vi "Untitled 5.vi"(2 "Camera Device  IN":T2, 3 "Camera Parameters":refnum<vi>, 4 "Selector":refnum<vi>, 5 "Stream?":refnum<vi>) -> (0 "Stream? OUT":bool, 1 "Camera Device OUT":T1)   [LabVIEW 2010]
uses:
  <vilib>/addons/PixeLINK/Low Level Functions/CAMERA_FEATURES.llb/TDPU-CameraFeatures-PixelFormat.ctl
  <vilib>/addons/PixeLINK/Low Level Functions/CAMERA_FEATURES.llb/TDPU-CameraFeatures-FeatureFlags.ctl
  <vilib>/addons/PixeLINK/Low Level Functions/CAMERA_FEATURES.llb/TDPU-CameraFeatures-FeatureIds.ctl
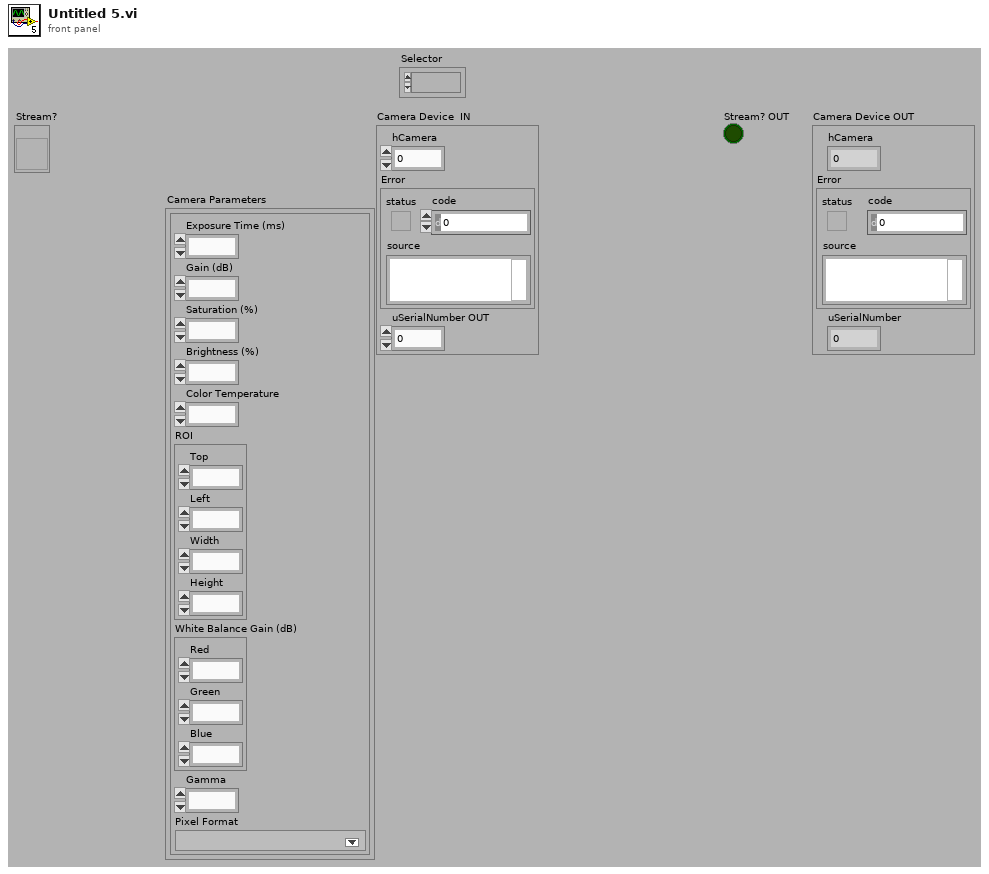
[diagram p1: front panel]
types:
  T1 = cluster{"hCamera":u32, "Error":errorcluster, "uSerialNumber":u32}
  T2 = cluster{"hCamera":u32, "Error":errorcluster, "uSerialNumber OUT":u32}
  T3 = typedef "TDPU-CameraFeatures-PixelFormat.ctl" = u16
  T4 = cluster{"Selector":u16, "Stream?":bool, "Camera Parameters":cluster{"Exposure Time (ms)":u32, "Gain (dB)":dbl, "Saturation (%)":dbl, "Brightness (%)":dbl, "Color Temperature":dbl, "ROI":cluster{"Top":i32, "Left":i32, "Width":i32, "Height":i32}, "White Balance Gain (dB)":cluster{"Red":dbl, "Green":dbl, "Blue":dbl}, "Gamma":dbl, "Pixel Format":T3}}
  T5 = cluster{"Exposure Time (ms)":u32, "Gain (dB)":dbl, "Saturation (%)":dbl, "Brightness (%)":dbl, "Color Temperature":dbl, "ROI":cluster{"Top":i32, "Left":i32, "Width":i32, "Height":i32}, "White Balance Gain (dB)":cluster{"Red":dbl, "Green":dbl, "Blue":dbl}, "Gamma":dbl, "Pixel Format":T3}
  T6 = cluster{"Exposure Time (ms)":dbl, "Gain (dB)":dbl, "Saturation (%)":dbl, "Brightness (%)":dbl, "Color Temperature":dbl, "ROI":cluster{"Top":i32, "Left":i32, "Width":i32, "Height":i32}, "White Balance Gain (dB)":cluster{"Red":dbl, "Green":dbl, "Blue":dbl}, "Gamma":dbl, "Pixel Format":T3}
  T7 = enum16{"Exposure Time (ms)", "Gain (dB)", "Saturation (%)", "Brightness (%)", "Color Temperature (%)", "ROI", "White Balance Gain (dB)", "Gamma", "Pixel Format", "Selector", "Stream", "Nothing"}[]
  T8 = typedef "TDPU-CameraFeatures-FeatureFlags.ctl" = u32
  T9 = typedef "TDPU-CameraFeatures-FeatureIds.ctl" = u32
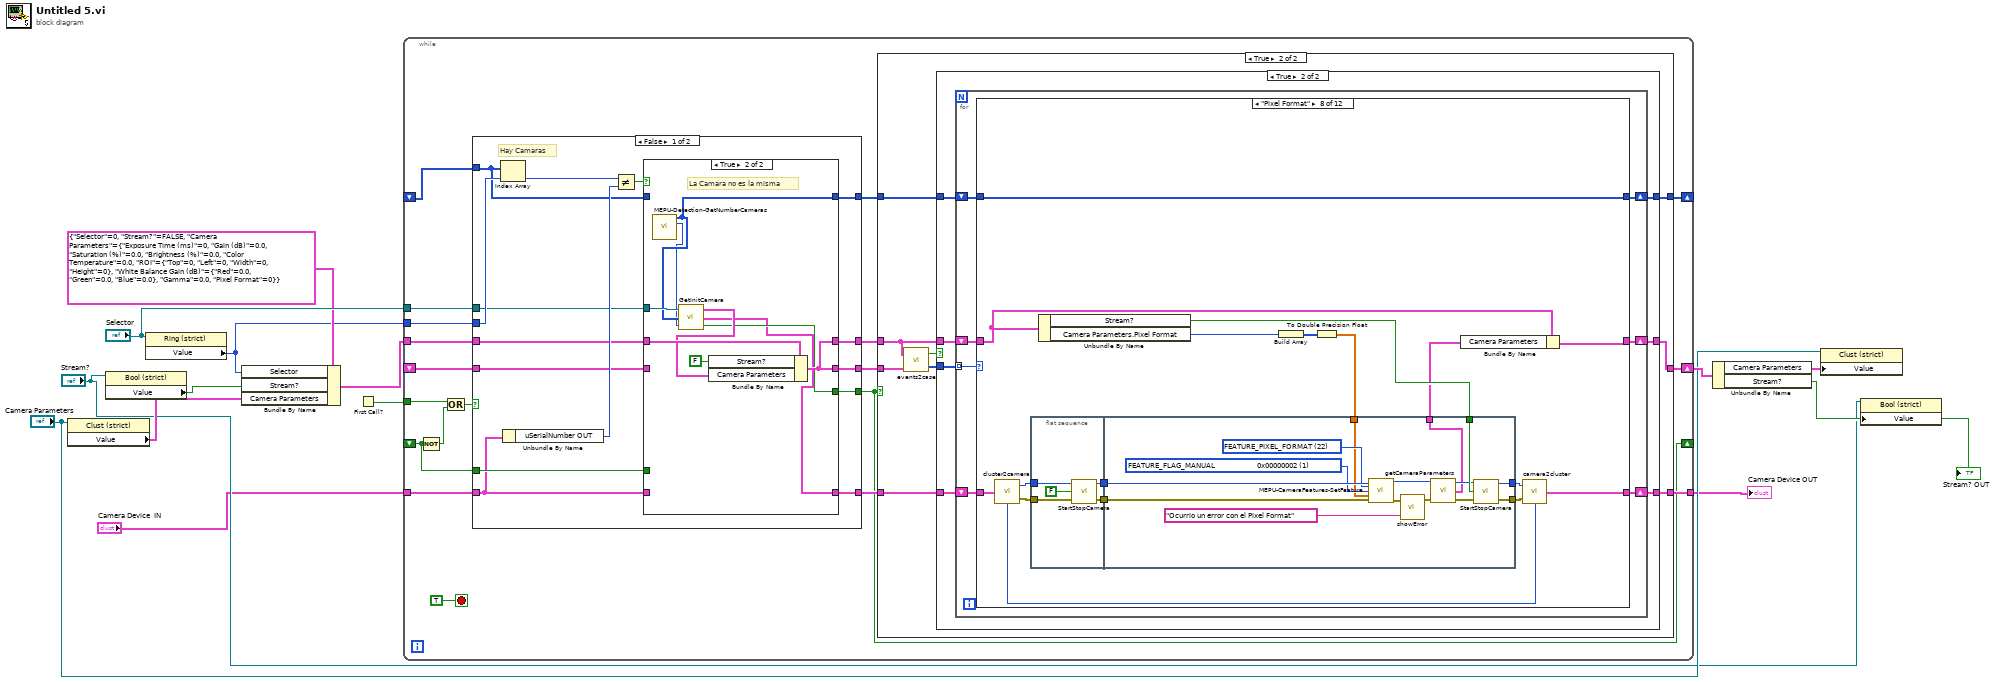
[diagram p0: block diagram]
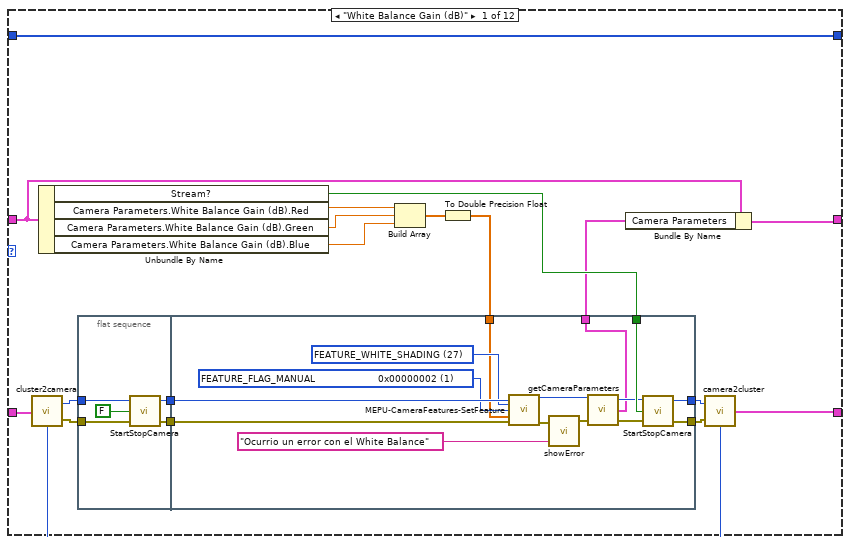
[diagram p4: hidden frame]
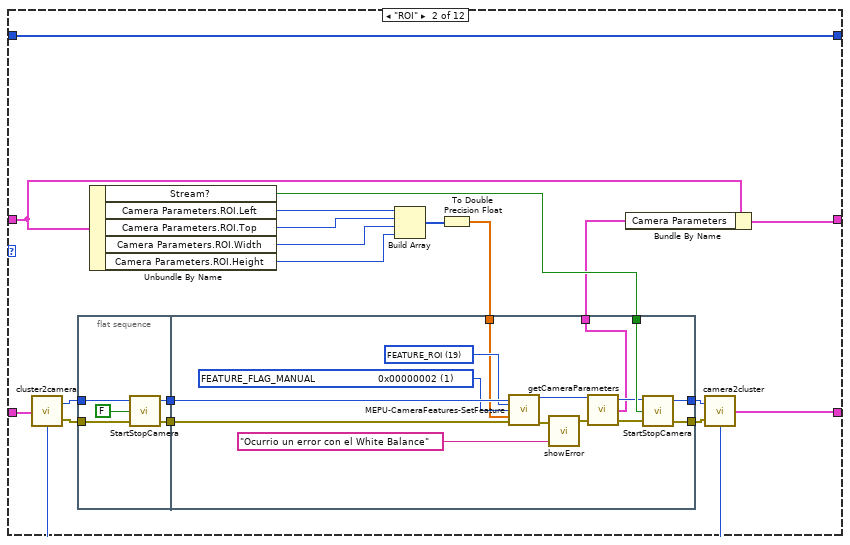
[diagram p5: hidden frame]
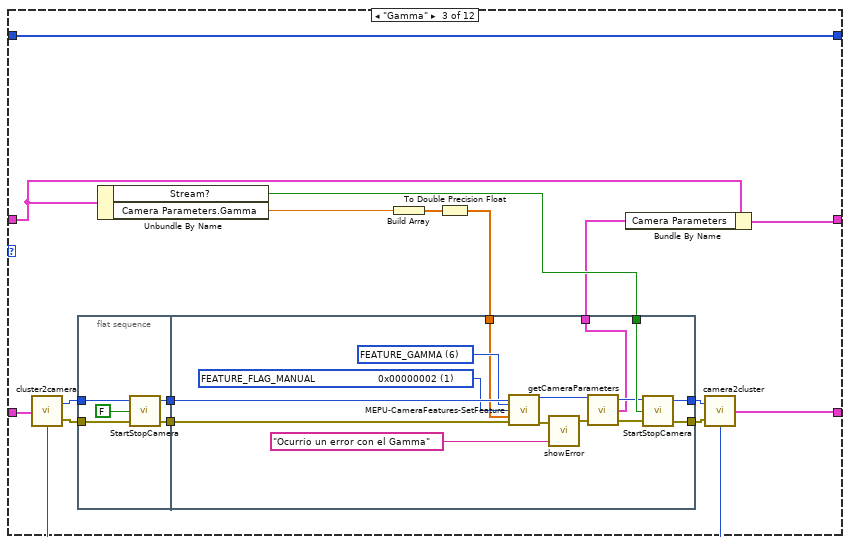
[diagram p6: hidden frame]
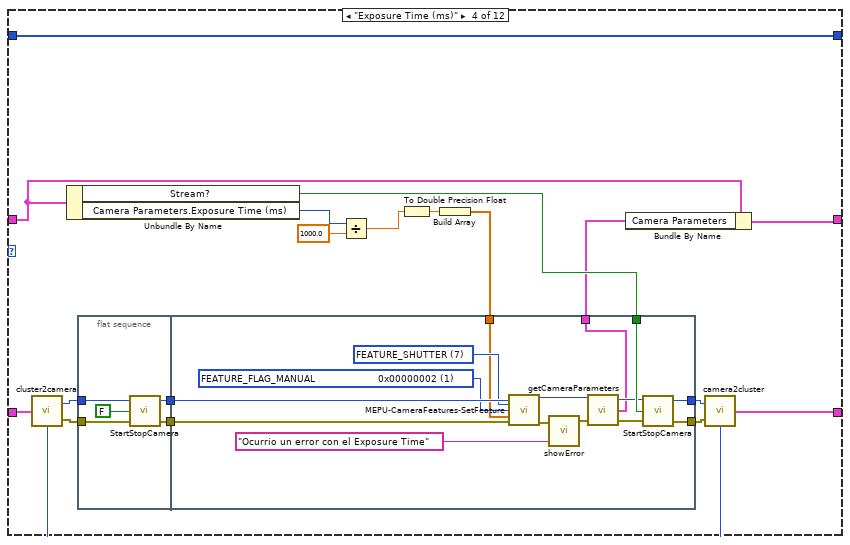
[diagram p7: hidden frame]
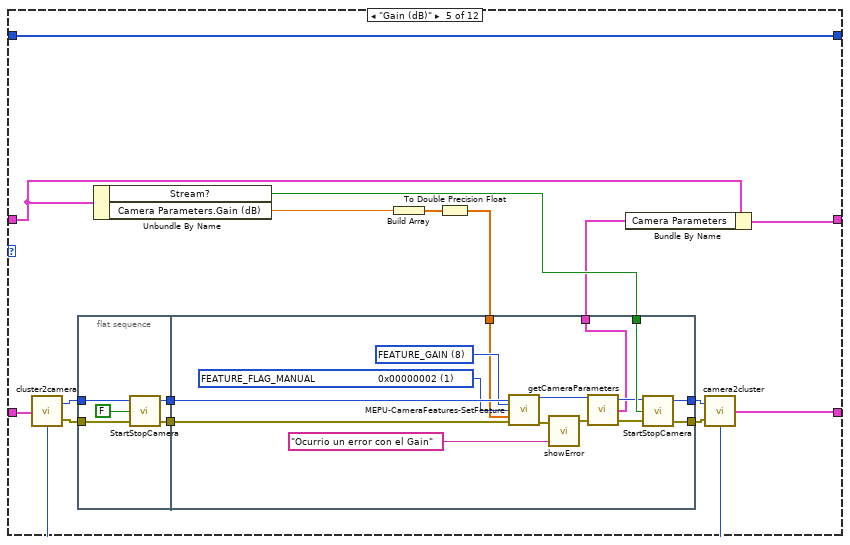
[diagram p8: hidden frame]
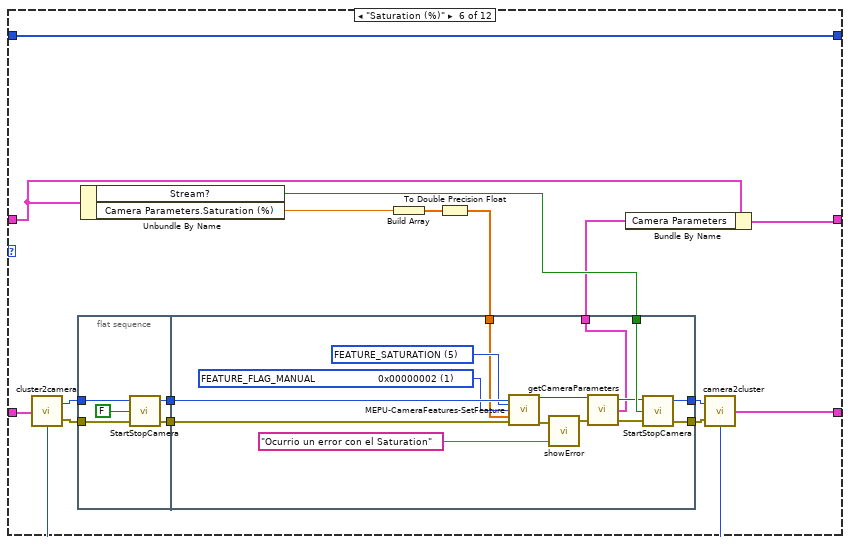
[diagram p9: hidden frame]
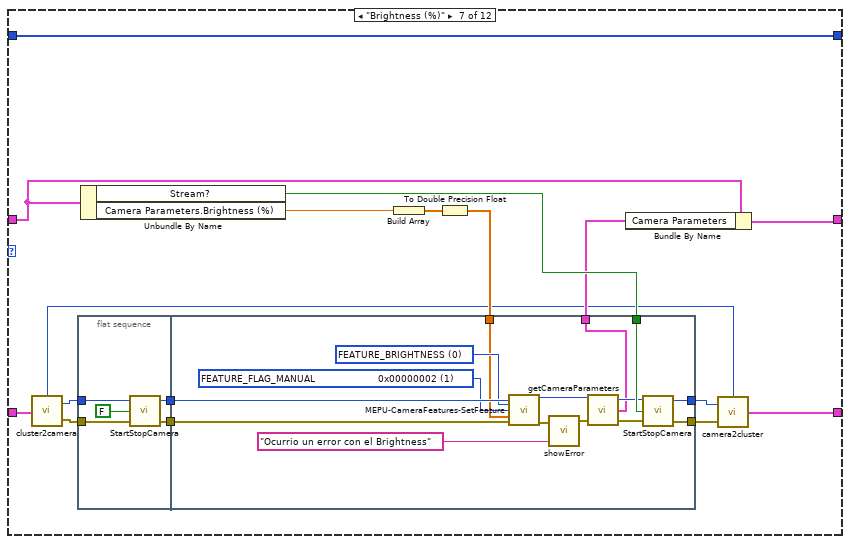
[diagram p10: hidden frame]
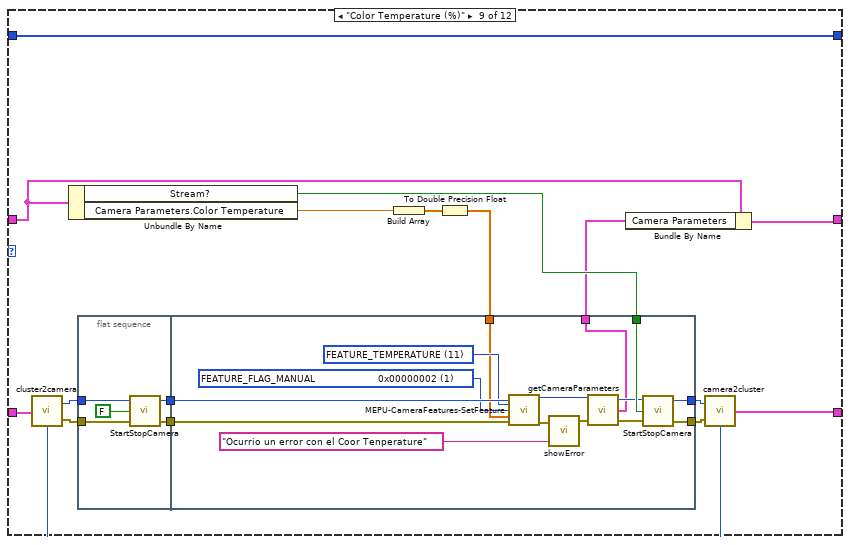
[diagram p11: hidden frame]
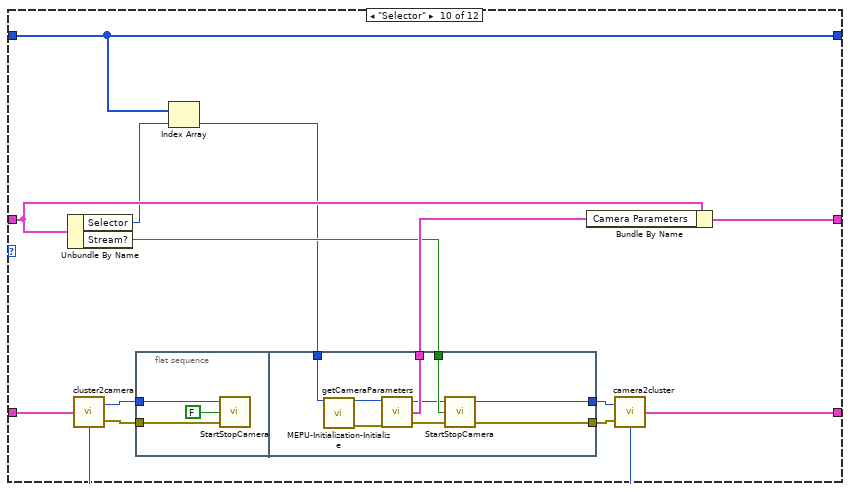
[diagram p12: hidden frame]
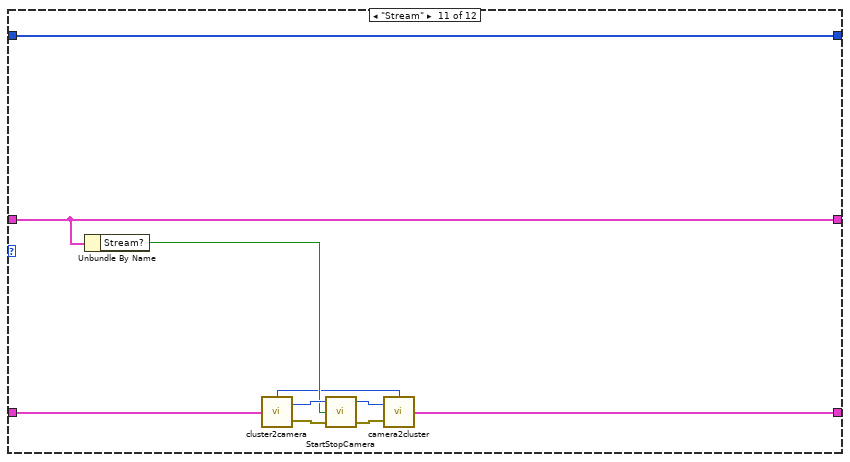
[diagram p13: hidden frame]
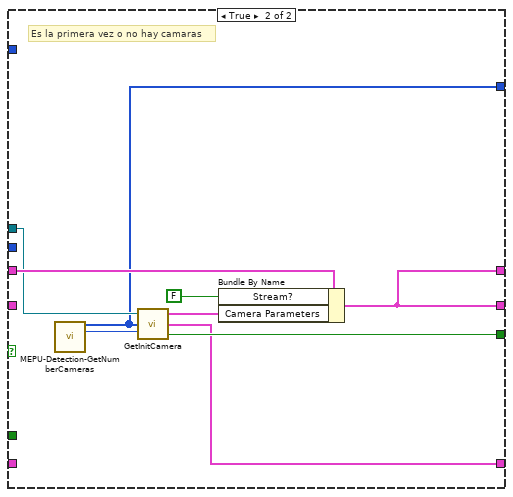
[diagram p16: hidden frame]
diagram:
  n1 = property class="Clust (strict)"(reference="Camera Parameters") -> ("Value"=w7:T5)  [unwired: 1 in, 2 out]
  n2 = property class="Bool (strict)"(reference="Stream?") -> ("Value"=w6:bool)  [unwired: 1 in, 2 out]
  n3 = property class="Ring (strict)"(reference="Selector") -> ("Value"=w3:u16)  [unwired: 1 in, 2 out]
  n4 = Bundle By Name(cluster=T4 {"Selector"=0, "Stream?"=FALSE, "Camera Parameters"={"Exposure Time (ms)"=0, "Gain (dB)"=0.0, "Saturation (%)"=0.0, "Brightness (%)"=0.0, "Color Temperature"=0.0, "ROI"={"Top"=0, "Left"=0, "Width"=0, "Height"=0}, "White Balance Gain (dB)"={"Red"=0.0, "Green"=0.0, "Blue"=0.0}, "Gamma"=0.0, "Pixel Format"=0}}, "Selector"=w3, "Stream?"=w6, "Camera Parameters"=w7) -> (w13:T4)
  n5 = First Call?() -> (First Call?: T/F=w14:bool)
  n6 = while {
    tunnel: w13 -> [w29]
    shift-right: [w32] -> w12
    shift-left: _ -> [w28]
    tunnel: "Camera Device  IN" -> [w25]
    tunnel: [w31] -> w1
    tunnel: w14 -> [w18]
    tunnel: "Selector" -> [w24]
    shift-right: [w20] -> _
    shift-left: _ -> [w23]
    shift-right: [w19] -> _
    shift-left: _ -> [w15]
    tunnel: w3 -> [w16]
    stop <- TRUE stop-if-true
    n7 = Not(x=w15) -> (.not. x?=w17:bool)
    n8 = Or(x=w18, y=w17) -> (x .or. y?=w22:bool)
    n9 = case shown="False" w22 {
      tunnel: [w452 w475] -> w21
      tunnel: [w450 w478] -> w30
      tunnel: w29 -> [w449 w479]
      tunnel: w28 -> [w447 _]
      tunnel: [w448 w478] -> w27
      tunnel: [w444 w471] -> w26
      tunnel: w25 -> [w443 _]
      tunnel: w23 -> [w451 _]
      tunnel: [w446 w473] -> w19
      tunnel: w24 -> [w442 w476]
      tunnel: w16 -> [w456 _]
      tunnel: w15 -> [w445 _]
      frame False {
        # "Hay Camaras"
        n10 = Index Array(array=w451, index=w456) -> (element=w455:u32)
        n11 = Unbundle By Name(w443) -> ("uSerialNumber OUT"=w454:u32)
        n12 = Not Equal?(x=w455, y=w454) -> (x != y?=w453:bool)
        n13 = case shown="True" w453 {
          tunnel: [w461 w469] -> w452
          tunnel: w451 -> [w461 _]
          tunnel: [w460 w466] -> w450
          tunnel: w449 -> [w460 w467]
          tunnel: [w459 w466] -> w448
          tunnel: w447 -> [w459 _]
          tunnel: [w458 w463] -> w446
          tunnel: w445 -> [w458 _]
          tunnel: [w457 w462] -> w444
          tunnel: w443 -> [w457 _]
          tunnel: w442 -> [_ w470]
          frame False {
            # "Sigue siendo todo igual"
          }
          frame True {
            # "La Camara no es la misma"
            n14 = call <vilib>:"MEPU-Detection-GetNumberCameras.vi"() -> ("LV_SerialNumbers OUT"=w469:u32[], "LV_NumberSerial OUT"=w468:u32)  [unwired: 13 in, 1 out]
            n15 = call "GetInitCamera.vi"("LV_NumberSerial IN"=w468, "LV_SerialNumbers IN"=w469, "Selector"=w470) -> ("Hay Camaras?"=w463:bool, "Camera Device OUT"=w462:T2, "Camera Parameters OUT"=w464:T6)
            n16 = Bundle By Name(cluster=w467, "Stream?"=FALSE, "Camera Parameters"=w464) -> (w466:T4)
          }
        }
      }
      frame True {
        # "Es la primera vez o no hay camaras"
        n17 = call <vilib>:"MEPU-Detection-GetNumberCameras.vi"() -> ("LV_SerialNumbers OUT"=w475:u32[], "LV_NumberSerial OUT"=w474:u32)  [unwired: 13 in, 1 out]
        n18 = call "GetInitCamera.vi"("LV_NumberSerial IN"=w474, "LV_SerialNumbers IN"=w475, "Selector"=w476) -> ("Hay Camaras?"=w473:bool, "Camera Device OUT"=w471:T2, "Camera Parameters OUT"=w472:T6)
        n19 = Bundle By Name(cluster=w479, "Stream?"=FALSE, "Camera Parameters"=w472) -> (w478:T4)
      }
    }
    n20 = case shown="True" w19 {
      tunnel: [w36 w44] -> w32
      tunnel: [w35 w42] -> w31
      tunnel: w21 -> [w34 w41]
      tunnel: w30 -> [w36 w40]
      tunnel: w27 -> [_ w39]
      tunnel: w26 -> [w35 w38]
      tunnel: [w34 w37] -> w20
      frame False {
      }
      frame True {
        n21 = call "events2case.vi"("Controls Old"=w39, "Controls New"=w40) -> ("Cambios"=w43:T7, "Cambio?"=w45:bool)
        n22 = case shown="True" w45 {
          tunnel: [w48 w53] -> w44
          tunnel: w40 -> [w48 w54]
          tunnel: w43 -> [_ w55]
          tunnel: w38 -> [w47 w52]
          tunnel: [w47 w51] -> w42
          tunnel: w41 -> [w46 w50]
          tunnel: [w46 w49] -> w37
          frame False {
          }
          frame True {
            n23 = for {
              tunnel: w55 -> [w62] mode=indexing
              shift-right: [w60] -> w53
              shift-left: w54 -> [w61]
              shift-right: [w58] -> w51
              shift-left: w52 -> [w59]
              shift-right: [w57] -> w49
              shift-left: w50 -> [w56]
              n24 = case shown="\"Pixel Format\"" w62 {
                tunnel: w61 -> [w73 w113 w150 w189 w226 w263 w302 w337 w374 w415 w437 w441]
                tunnel: [w74 w114 w151 w190 w227 w264 w303 w338 w375 w416 w437 w441] -> w60
                tunnel: w59 -> [w65 w102 w144 w180 w219 w256 w293 w330 w368 w405 w431 w440]
                tunnel: [w64 w103 w143 w181 w220 w257 w294 w331 w366 w404 w430 w440] -> w58
                tunnel: [w68 w108 w147 w187 w223 w260 w299 w334 w371 w409 w438 w439] -> w57
                tunnel: w56 -> [w68 w108 w147 w187 w223 w260 w299 w334 w371 w409 w438 w439]
                frame "White Balance Gain (dB)" {
                  n25 = call "cluster2camera.vi"("Camera Device IN"=w65) -> ("Error OUT"=w78:errorcluster, "hCamera OUT"=w79:u32, "uSerialNumber OUT"=w63:u32)  [unwired: 2 in]
                  n26 = Unbundle By Name(w73) -> ("Stream?"=w75:bool, "Camera Parameters.White Balance Gain (dB).Red"=w72:dbl, "Camera Parameters.White Balance Gain (dB).Green"=w71:dbl, "Camera Parameters.White Balance Gain (dB).Blue"=w70:dbl)
                  n27 = flat-sequence {
                    tunnel: w79 -> [w85]
                    tunnel: w78 -> [w84]
                    tunnel: [w83] -> w81
                    tunnel: [w82] -> w80
                    tunnel: w75 -> [w101]
                    tunnel: [w100] -> w77
                    tunnel: [w99] -> w76
                    tunnel: w81 -> [w98]
                    tunnel: w80 -> [w97]
                    tunnel: [w91] -> w69
                    tunnel: w66 -> [w90]
                    frame #0 {
                      n28 = call "StartStopCamera.vi"("Error IN"=w84, "Camara ON?"=FALSE, "hCamera IN"=w85) -> ("Error OUT"=w82:errorcluster, "hCamera OUT"=w83:u32)  [unwired: 1 in]
                    }
                    frame #1 {
                      w95 = T8 1 items=["FEATURE_FLAG_PRESENCE                 0x00000001", "FEATURE_FLAG_MANUAL                     0x00000002", "FEATURE_FLAG_AUTO                         0x00000004", "FEATURE_FLAG_ONEPUSH                   0x00000008", "FEATURE_FLAG_OFF                            0x00000010", "FEATURE_FLAG_DESC_SUPPORTED    0x00000020", "FEATURE_FLAG_READ_ONLY               0x00000040"] ("uFlags IN")
                      w96 = T9 27 items=["FEATURE_BRIGHTNESS", "FEATURE_EXPOSURE", "FEATURE_SHARPNESS", "FEATURE_WHITE_BAL", "FEATURE_HUE", "FEATURE_SATURATION", "FEATURE_GAMMA", "FEATURE_SHUTTER", "FEATURE_GAIN", "FEATURE_IRIS", "FEATURE_FOCUS", "FEATURE_TEMPERATURE", "FEATURE_TRIGGER", "FEATURE_ZOOM", "FEATURE_PAN", "FEATURE_TILT", "FEATURE_OPT_FILTER", "FEATURE_GPIO", "FEATURE_FRAME_RATE", "FEATURE_ROI", "FEATURE_FLIP", "FEATURE_PIXEL_ADDRESSING", "FEATURE_PIXEL_FORMAT", "FEATURE_EXTENDED_SHUTTER", "FEATURE_AUTO_ROI", "FEATURE_LOOKUP_TABLE", "FEATURE_MEMORY_CHANNEL", "FEATURE_WHITE_SHADING", "FEATURE_ROTATE", "FEATURE_IMAGER_CLK_DIVISOR", "FEATURE_TRIG_WITH_CNTRLD_LIGHT", "FEATURE_MAX_PIXEL_SIZE"] ("uFeatureId IN")
                      n29 = call <vilib>:"MEPU-CameraFeatures-SetFeature.vi"("hCamera IN"=w98, "uFeatureId IN"=w96, "uFlags IN"=w95, "pParms IN"=w90, "Error IN"=w97) -> ("hCamera OUT"=w94:u32, "Error OUT"=w89:errorcluster)  [unwired: 8 in, 1 out]
                      n30 = call "showError.vi"("message"="Ocurrio un error con el White Balance", "Error IN"=w89) -> ("Error OUT"=w88:errorcluster)  [unwired: 3 in]
                      n31 = call "getCameraParameters.vi"("Error IN"=w88, "hCamera IN"=w94) -> ("Error OUT"=w92:errorcluster, "Camera Parameters"=w91:T6, "hCamera OUT"=w93:u32)  [unwired: 1 in]
                      n32 = call "StartStopCamera.vi"("Error IN"=w92, "Camara ON?"=w101, "hCamera IN"=w93) -> ("Error OUT"=w99:errorcluster, "hCamera OUT"=w100:u32)  [unwired: 1 in]
                    }
                  }
                  n33 = Build Array(w72, w71, w70) -> (w67:dbl[])
                  n34 = To Double Precision Float(number=w67) -> (double precision float=w66:dbl[])
                  n35 = Bundle By Name(cluster=w73, "Camera Parameters"=w69) -> (w74:T4)
                  n36 = call "camera2cluster.vi"("uSerialNumber IN"=w63, "Error IN"=w76, "hCamera IN"=w77) -> ("Camera Device OUT"=w64:T1)
                }
                frame "ROI" {
                  n37 = call "cluster2camera.vi"("Camera Device IN"=w102) -> ("Error OUT"=w118:errorcluster, "hCamera OUT"=w119:u32, "uSerialNumber OUT"=w104:u32)  [unwired: 2 in]
                  n38 = flat-sequence {
                    tunnel: w119 -> [w125]
                    tunnel: w118 -> [w124]
                    tunnel: [w123] -> w121
                    tunnel: [w122] -> w120
                    tunnel: w115 -> [w141]
                    tunnel: [w140] -> w117
                    tunnel: [w139] -> w116
                    tunnel: w121 -> [w138]
                    tunnel: w120 -> [w137]
                    tunnel: [w131] -> w109
                    tunnel: w105 -> [w130]
                    frame #0 {
                      n39 = call "StartStopCamera.vi"("Error IN"=w124, "Camara ON?"=FALSE, "hCamera IN"=w125) -> ("Error OUT"=w122:errorcluster, "hCamera OUT"=w123:u32)  [unwired: 1 in]
                    }
                    frame #1 {
                      w135 = T8 1 items=["FEATURE_FLAG_PRESENCE                 0x00000001", "FEATURE_FLAG_MANUAL                     0x00000002", "FEATURE_FLAG_AUTO                         0x00000004", "FEATURE_FLAG_ONEPUSH                   0x00000008", "FEATURE_FLAG_OFF                            0x00000010", "FEATURE_FLAG_DESC_SUPPORTED    0x00000020", "FEATURE_FLAG_READ_ONLY               0x00000040"] ("uFlags IN")
                      w136 = T9 19 items=["FEATURE_BRIGHTNESS", "FEATURE_EXPOSURE", "FEATURE_SHARPNESS", "FEATURE_WHITE_BAL", "FEATURE_HUE", "FEATURE_SATURATION", "FEATURE_GAMMA", "FEATURE_SHUTTER", "FEATURE_GAIN", "FEATURE_IRIS", "FEATURE_FOCUS", "FEATURE_TEMPERATURE", "FEATURE_TRIGGER", "FEATURE_ZOOM", "FEATURE_PAN", "FEATURE_TILT", "FEATURE_OPT_FILTER", "FEATURE_GPIO", "FEATURE_FRAME_RATE", "FEATURE_ROI", "FEATURE_FLIP", "FEATURE_PIXEL_ADDRESSING", "FEATURE_PIXEL_FORMAT", "FEATURE_EXTENDED_SHUTTER", "FEATURE_AUTO_ROI", "FEATURE_LOOKUP_TABLE", "FEATURE_MEMORY_CHANNEL", "FEATURE_WHITE_SHADING", "FEATURE_ROTATE", "FEATURE_IMAGER_CLK_DIVISOR", "FEATURE_TRIG_WITH_CNTRLD_LIGHT", "FEATURE_MAX_PIXEL_SIZE"] ("uFeatureId IN")
                      n40 = call <vilib>:"MEPU-CameraFeatures-SetFeature.vi"("hCamera IN"=w138, "uFeatureId IN"=w136, "uFlags IN"=w135, "pParms IN"=w130, "Error IN"=w137) -> ("hCamera OUT"=w134:u32, "Error OUT"=w129:errorcluster)  [unwired: 8 in, 1 out]
                      n41 = call "showError.vi"("message"="Ocurrio un error con el White Balance", "Error IN"=w129) -> ("Error OUT"=w128:errorcluster)  [unwired: 3 in]
                      n42 = call "getCameraParameters.vi"("Error IN"=w128, "hCamera IN"=w134) -> ("Error OUT"=w132:errorcluster, "Camera Parameters"=w131:T6, "hCamera OUT"=w133:u32)  [unwired: 1 in]
                      n43 = call "StartStopCamera.vi"("Error IN"=w132, "Camara ON?"=w141, "hCamera IN"=w133) -> ("Error OUT"=w139:errorcluster, "hCamera OUT"=w140:u32)  [unwired: 1 in]
                    }
                  }
                  n44 = Unbundle By Name(w113) -> ("Stream?"=w115:bool, "Camera Parameters.ROI.Left"=w112:i32, "Camera Parameters.ROI.Top"=w111:i32, "Camera Parameters.ROI.Width"=w110:i32, "Camera Parameters.ROI.Height"=w107:i32)
                  n45 = Build Array(w112, w111, w110, w107) -> (w106:i32[])
                  n46 = To Double Precision Float(number=w106) -> (double precision float=w105:dbl[])
                  n47 = Bundle By Name(cluster=w113, "Camera Parameters"=w109) -> (w114:T4)
                  n48 = call "camera2cluster.vi"("uSerialNumber IN"=w104, "Error IN"=w116, "hCamera IN"=w117) -> ("Camera Device OUT"=w103:T1)
                }
                frame "Gamma" {
                  n49 = call "cluster2camera.vi"("Camera Device IN"=w144) -> ("Error OUT"=w155:errorcluster, "hCamera OUT"=w156:u32, "uSerialNumber OUT"=w142:u32)  [unwired: 2 in]
                  n50 = flat-sequence {
                    tunnel: w156 -> [w162]
                    tunnel: w155 -> [w161]
                    tunnel: [w160] -> w158
                    tunnel: [w159] -> w157
                    tunnel: w152 -> [w178]
                    tunnel: [w177] -> w154
                    tunnel: [w176] -> w153
                    tunnel: w158 -> [w175]
                    tunnel: w157 -> [w174]
                    tunnel: [w168] -> w148
                    tunnel: w145 -> [w167]
                    frame #0 {
                      n51 = call "StartStopCamera.vi"("Error IN"=w161, "Camara ON?"=FALSE, "hCamera IN"=w162) -> ("Error OUT"=w159:errorcluster, "hCamera OUT"=w160:u32)  [unwired: 1 in]
                    }
                    frame #1 {
                      w172 = T8 1 items=["FEATURE_FLAG_PRESENCE                 0x00000001", "FEATURE_FLAG_MANUAL                     0x00000002", "FEATURE_FLAG_AUTO                         0x00000004", "FEATURE_FLAG_ONEPUSH                   0x00000008", "FEATURE_FLAG_OFF                            0x00000010", "FEATURE_FLAG_DESC_SUPPORTED    0x00000020", "FEATURE_FLAG_READ_ONLY               0x00000040"] ("uFlags IN")
                      w173 = T9 6 items=["FEATURE_BRIGHTNESS", "FEATURE_EXPOSURE", "FEATURE_SHARPNESS", "FEATURE_WHITE_BAL", "FEATURE_HUE", "FEATURE_SATURATION", "FEATURE_GAMMA", "FEATURE_SHUTTER", "FEATURE_GAIN", "FEATURE_IRIS", "FEATURE_FOCUS", "FEATURE_TEMPERATURE", "FEATURE_TRIGGER", "FEATURE_ZOOM", "FEATURE_PAN", "FEATURE_TILT", "FEATURE_OPT_FILTER", "FEATURE_GPIO", "FEATURE_FRAME_RATE", "FEATURE_ROI", "FEATURE_FLIP", "FEATURE_PIXEL_ADDRESSING", "FEATURE_PIXEL_FORMAT", "FEATURE_EXTENDED_SHUTTER", "FEATURE_AUTO_ROI", "FEATURE_LOOKUP_TABLE", "FEATURE_MEMORY_CHANNEL", "FEATURE_WHITE_SHADING", "FEATURE_ROTATE", "FEATURE_IMAGER_CLK_DIVISOR", "FEATURE_TRIG_WITH_CNTRLD_LIGHT", "FEATURE_MAX_PIXEL_SIZE"] ("uFeatureId IN")
                      n52 = call <vilib>:"MEPU-CameraFeatures-SetFeature.vi"("hCamera IN"=w175, "uFeatureId IN"=w173, "uFlags IN"=w172, "pParms IN"=w167, "Error IN"=w174) -> ("hCamera OUT"=w171:u32, "Error OUT"=w166:errorcluster)  [unwired: 8 in, 1 out]
                      n53 = call "showError.vi"("message"="Ocurrio un error con el Gamma", "Error IN"=w166) -> ("Error OUT"=w165:errorcluster)  [unwired: 3 in]
                      n54 = call "getCameraParameters.vi"("Error IN"=w165, "hCamera IN"=w171) -> ("Error OUT"=w169:errorcluster, "Camera Parameters"=w168:T6, "hCamera OUT"=w170:u32)  [unwired: 1 in]
                      n55 = call "StartStopCamera.vi"("Error IN"=w169, "Camara ON?"=w178, "hCamera IN"=w170) -> ("Error OUT"=w176:errorcluster, "hCamera OUT"=w177:u32)  [unwired: 1 in]
                    }
                  }
                  n56 = Unbundle By Name(w150) -> ("Stream?"=w152:bool, "Camera Parameters.Gamma"=w149:dbl)
                  n57 = Build Array(w149) -> (w146:dbl[])
                  n58 = To Double Precision Float(number=w146) -> (double precision float=w145:dbl[])
                  n59 = Bundle By Name(cluster=w150, "Camera Parameters"=w148) -> (w151:T4)
                  n60 = call "camera2cluster.vi"("uSerialNumber IN"=w142, "Error IN"=w153, "hCamera IN"=w154) -> ("Camera Device OUT"=w143:T1)
                }
                frame "Exposure Time (ms)" {
                  n61 = call "cluster2camera.vi"("Camera Device IN"=w180) -> ("Error OUT"=w194:errorcluster, "hCamera OUT"=w195:u32, "uSerialNumber OUT"=w179:u32)  [unwired: 2 in]
                  n62 = Unbundle By Name(w189) -> ("Stream?"=w191:bool, "Camera Parameters.Exposure Time (ms)"=w186:u32)
                  n63 = flat-sequence {
                    tunnel: w195 -> [w201]
                    tunnel: w194 -> [w200]
                    tunnel: [w199] -> w197
                    tunnel: [w198] -> w196
                    tunnel: w191 -> [w217]
                    tunnel: [w216] -> w193
                    tunnel: [w215] -> w192
                    tunnel: w197 -> [w214]
                    tunnel: w196 -> [w213]
                    tunnel: [w207] -> w188
                    tunnel: w184 -> [w206]
                    frame #0 {
                      n64 = call "StartStopCamera.vi"("Error IN"=w200, "Camara ON?"=FALSE, "hCamera IN"=w201) -> ("Error OUT"=w198:errorcluster, "hCamera OUT"=w199:u32)  [unwired: 1 in]
                    }
                    frame #1 {
                      w211 = T8 1 items=["FEATURE_FLAG_PRESENCE                 0x00000001", "FEATURE_FLAG_MANUAL                     0x00000002", "FEATURE_FLAG_AUTO                         0x00000004", "FEATURE_FLAG_ONEPUSH                   0x00000008", "FEATURE_FLAG_OFF                            0x00000010", "FEATURE_FLAG_DESC_SUPPORTED    0x00000020", "FEATURE_FLAG_READ_ONLY               0x00000040"] ("uFlags IN")
                      w212 = T9 7 items=["FEATURE_BRIGHTNESS", "FEATURE_EXPOSURE", "FEATURE_SHARPNESS", "FEATURE_WHITE_BAL", "FEATURE_HUE", "FEATURE_SATURATION", "FEATURE_GAMMA", "FEATURE_SHUTTER", "FEATURE_GAIN", "FEATURE_IRIS", "FEATURE_FOCUS", "FEATURE_TEMPERATURE", "FEATURE_TRIGGER", "FEATURE_ZOOM", "FEATURE_PAN", "FEATURE_TILT", "FEATURE_OPT_FILTER", "FEATURE_GPIO", "FEATURE_FRAME_RATE", "FEATURE_ROI", "FEATURE_FLIP", "FEATURE_PIXEL_ADDRESSING", "FEATURE_PIXEL_FORMAT", "FEATURE_EXTENDED_SHUTTER", "FEATURE_AUTO_ROI", "FEATURE_LOOKUP_TABLE", "FEATURE_MEMORY_CHANNEL", "FEATURE_WHITE_SHADING", "FEATURE_ROTATE", "FEATURE_IMAGER_CLK_DIVISOR", "FEATURE_TRIG_WITH_CNTRLD_LIGHT", "FEATURE_MAX_PIXEL_SIZE"] ("uFeatureId IN")
                      n65 = call <vilib>:"MEPU-CameraFeatures-SetFeature.vi"("hCamera IN"=w214, "uFeatureId IN"=w212, "uFlags IN"=w211, "pParms IN"=w206, "Error IN"=w213) -> ("hCamera OUT"=w210:u32, "Error OUT"=w205:errorcluster)  [unwired: 8 in, 1 out]
                      n66 = call "showError.vi"("message"="Ocurrio un error con el Exposure Time", "Error IN"=w205) -> ("Error OUT"=w204:errorcluster)  [unwired: 3 in]
                      n67 = call "getCameraParameters.vi"("Error IN"=w204, "hCamera IN"=w210) -> ("Error OUT"=w208:errorcluster, "Camera Parameters"=w207:T6, "hCamera OUT"=w209:u32)  [unwired: 1 in]
                      n68 = call "StartStopCamera.vi"("Error IN"=w208, "Camara ON?"=w217, "hCamera IN"=w209) -> ("Error OUT"=w215:errorcluster, "hCamera OUT"=w216:u32)  [unwired: 1 in]
                    }
                  }
                  n69 = Divide(x=w186, y=1000.0) -> (x/y=w183:dbl)
                  n70 = To Double Precision Float(number=w183) -> (double precision float=w182:dbl)
                  n71 = Build Array(w182) -> (w184:dbl[])
                  n72 = Bundle By Name(cluster=w189, "Camera Parameters"=w188) -> (w190:T4)
                  n73 = call "camera2cluster.vi"("uSerialNumber IN"=w179, "Error IN"=w192, "hCamera IN"=w193) -> ("Camera Device OUT"=w181:T1)
                }
                frame "Gain (dB)" {
                  n74 = call "cluster2camera.vi"("Camera Device IN"=w219) -> ("Error OUT"=w231:errorcluster, "hCamera OUT"=w232:u32, "uSerialNumber OUT"=w218:u32)  [unwired: 2 in]
                  n75 = flat-sequence {
                    tunnel: w232 -> [w238]
                    tunnel: w231 -> [w237]
                    tunnel: [w236] -> w234
                    tunnel: [w235] -> w233
                    tunnel: w228 -> [w254]
                    tunnel: [w253] -> w230
                    tunnel: [w252] -> w229
                    tunnel: w234 -> [w251]
                    tunnel: w233 -> [w250]
                    tunnel: [w244] -> w224
                    tunnel: w221 -> [w243]
                    frame #0 {
                      n76 = call "StartStopCamera.vi"("Error IN"=w237, "Camara ON?"=FALSE, "hCamera IN"=w238) -> ("Error OUT"=w235:errorcluster, "hCamera OUT"=w236:u32)  [unwired: 1 in]
                    }
                    frame #1 {
                      w248 = T8 1 items=["FEATURE_FLAG_PRESENCE                 0x00000001", "FEATURE_FLAG_MANUAL                     0x00000002", "FEATURE_FLAG_AUTO                         0x00000004", "FEATURE_FLAG_ONEPUSH                   0x00000008", "FEATURE_FLAG_OFF                            0x00000010", "FEATURE_FLAG_DESC_SUPPORTED    0x00000020", "FEATURE_FLAG_READ_ONLY               0x00000040"] ("uFlags IN")
                      w249 = T9 8 items=["FEATURE_BRIGHTNESS", "FEATURE_EXPOSURE", "FEATURE_SHARPNESS", "FEATURE_WHITE_BAL", "FEATURE_HUE", "FEATURE_SATURATION", "FEATURE_GAMMA", "FEATURE_SHUTTER", "FEATURE_GAIN", "FEATURE_IRIS", "FEATURE_FOCUS", "FEATURE_TEMPERATURE", "FEATURE_TRIGGER", "FEATURE_ZOOM", "FEATURE_PAN", "FEATURE_TILT", "FEATURE_OPT_FILTER", "FEATURE_GPIO", "FEATURE_FRAME_RATE", "FEATURE_ROI", "FEATURE_FLIP", "FEATURE_PIXEL_ADDRESSING", "FEATURE_PIXEL_FORMAT", "FEATURE_EXTENDED_SHUTTER", "FEATURE_AUTO_ROI", "FEATURE_LOOKUP_TABLE", "FEATURE_MEMORY_CHANNEL", "FEATURE_WHITE_SHADING", "FEATURE_ROTATE", "FEATURE_IMAGER_CLK_DIVISOR", "FEATURE_TRIG_WITH_CNTRLD_LIGHT", "FEATURE_MAX_PIXEL_SIZE"] ("uFeatureId IN")
                      n77 = call <vilib>:"MEPU-CameraFeatures-SetFeature.vi"("hCamera IN"=w251, "uFeatureId IN"=w249, "uFlags IN"=w248, "pParms IN"=w243, "Error IN"=w250) -> ("hCamera OUT"=w247:u32, "Error OUT"=w242:errorcluster)  [unwired: 8 in, 1 out]
                      n78 = call "showError.vi"("message"="Ocurrio un error con el Gain", "Error IN"=w242) -> ("Error OUT"=w241:errorcluster)  [unwired: 3 in]
                      n79 = call "getCameraParameters.vi"("Error IN"=w241, "hCamera IN"=w247) -> ("Error OUT"=w245:errorcluster, "Camera Parameters"=w244:T6, "hCamera OUT"=w246:u32)  [unwired: 1 in]
                      n80 = call "StartStopCamera.vi"("Error IN"=w245, "Camara ON?"=w254, "hCamera IN"=w246) -> ("Error OUT"=w252:errorcluster, "hCamera OUT"=w253:u32)  [unwired: 1 in]
                    }
                  }
                  n81 = Unbundle By Name(w226) -> ("Stream?"=w228:bool, "Camera Parameters.Gain (dB)"=w225:dbl)
                  n82 = Build Array(w225) -> (w222:dbl[])
                  n83 = To Double Precision Float(number=w222) -> (double precision float=w221:dbl[])
                  n84 = Bundle By Name(cluster=w226, "Camera Parameters"=w224) -> (w227:T4)
                  n85 = call "camera2cluster.vi"("uSerialNumber IN"=w218, "Error IN"=w229, "hCamera IN"=w230) -> ("Camera Device OUT"=w220:T1)
                }
                frame "Saturation (%)" {
                  n86 = call "cluster2camera.vi"("Camera Device IN"=w256) -> ("Error OUT"=w268:errorcluster, "hCamera OUT"=w269:u32, "uSerialNumber OUT"=w255:u32)  [unwired: 2 in]
                  n87 = flat-sequence {
                    tunnel: w269 -> [w275]
                    tunnel: w268 -> [w274]
                    tunnel: [w273] -> w271
                    tunnel: [w272] -> w270
                    tunnel: w265 -> [w291]
                    tunnel: [w290] -> w267
                    tunnel: [w289] -> w266
                    tunnel: w271 -> [w288]
                    tunnel: w270 -> [w287]
                    tunnel: [w281] -> w261
                    tunnel: w258 -> [w280]
                    frame #0 {
                      n88 = call "StartStopCamera.vi"("Error IN"=w274, "Camara ON?"=FALSE, "hCamera IN"=w275) -> ("Error OUT"=w272:errorcluster, "hCamera OUT"=w273:u32)  [unwired: 1 in]
                    }
                    frame #1 {
                      w285 = T8 1 items=["FEATURE_FLAG_PRESENCE                 0x00000001", "FEATURE_FLAG_MANUAL                     0x00000002", "FEATURE_FLAG_AUTO                         0x00000004", "FEATURE_FLAG_ONEPUSH                   0x00000008", "FEATURE_FLAG_OFF                            0x00000010", "FEATURE_FLAG_DESC_SUPPORTED    0x00000020", "FEATURE_FLAG_READ_ONLY               0x00000040"] ("uFlags IN")
                      w286 = T9 5 items=["FEATURE_BRIGHTNESS", "FEATURE_EXPOSURE", "FEATURE_SHARPNESS", "FEATURE_WHITE_BAL", "FEATURE_HUE", "FEATURE_SATURATION", "FEATURE_GAMMA", "FEATURE_SHUTTER", "FEATURE_GAIN", "FEATURE_IRIS", "FEATURE_FOCUS", "FEATURE_TEMPERATURE", "FEATURE_TRIGGER", "FEATURE_ZOOM", "FEATURE_PAN", "FEATURE_TILT", "FEATURE_OPT_FILTER", "FEATURE_GPIO", "FEATURE_FRAME_RATE", "FEATURE_ROI", "FEATURE_FLIP", "FEATURE_PIXEL_ADDRESSING", "FEATURE_PIXEL_FORMAT", "FEATURE_EXTENDED_SHUTTER", "FEATURE_AUTO_ROI", "FEATURE_LOOKUP_TABLE", "FEATURE_MEMORY_CHANNEL", "FEATURE_WHITE_SHADING", "FEATURE_ROTATE", "FEATURE_IMAGER_CLK_DIVISOR", "FEATURE_TRIG_WITH_CNTRLD_LIGHT", "FEATURE_MAX_PIXEL_SIZE"] ("uFeatureId IN")
                      n89 = call <vilib>:"MEPU-CameraFeatures-SetFeature.vi"("hCamera IN"=w288, "uFeatureId IN"=w286, "uFlags IN"=w285, "pParms IN"=w280, "Error IN"=w287) -> ("hCamera OUT"=w284:u32, "Error OUT"=w279:errorcluster)  [unwired: 8 in, 1 out]
                      n90 = call "showError.vi"("message"="Ocurrio un error con el Saturation", "Error IN"=w279) -> ("Error OUT"=w278:errorcluster)  [unwired: 3 in]
                      n91 = call "getCameraParameters.vi"("Error IN"=w278, "hCamera IN"=w284) -> ("Error OUT"=w282:errorcluster, "Camera Parameters"=w281:T6, "hCamera OUT"=w283:u32)  [unwired: 1 in]
                      n92 = call "StartStopCamera.vi"("Error IN"=w282, "Camara ON?"=w291, "hCamera IN"=w283) -> ("Error OUT"=w289:errorcluster, "hCamera OUT"=w290:u32)  [unwired: 1 in]
                    }
                  }
                  n93 = Unbundle By Name(w263) -> ("Stream?"=w265:bool, "Camera Parameters.Saturation (%)"=w262:dbl)
                  n94 = Build Array(w262) -> (w259:dbl[])
                  n95 = To Double Precision Float(number=w259) -> (double precision float=w258:dbl[])
                  n96 = Bundle By Name(cluster=w263, "Camera Parameters"=w261) -> (w264:T4)
                  n97 = call "camera2cluster.vi"("uSerialNumber IN"=w255, "Error IN"=w266, "hCamera IN"=w267) -> ("Camera Device OUT"=w257:T1)
                }
                frame "Brightness (%)" {
                  n98 = call "cluster2camera.vi"("Camera Device IN"=w293) -> ("Error OUT"=w305:errorcluster, "hCamera OUT"=w306:u32, "uSerialNumber OUT"=w292:u32)  [unwired: 2 in]
                  n99 = flat-sequence {
                    tunnel: w306 -> [w312]
                    tunnel: w305 -> [w311]
                    tunnel: [w310] -> w308
                    tunnel: [w309] -> w307
                    tunnel: w304 -> [w328]
                    tunnel: [w327] -> w296
                    tunnel: [w326] -> w295
                    tunnel: w308 -> [w325]
                    tunnel: w307 -> [w324]
                    tunnel: [w318] -> w300
                    tunnel: w297 -> [w317]
                    frame #0 {
                      n100 = call "StartStopCamera.vi"("Error IN"=w311, "Camara ON?"=FALSE, "hCamera IN"=w312) -> ("Error OUT"=w309:errorcluster, "hCamera OUT"=w310:u32)  [unwired: 1 in]
                    }
                    frame #1 {
                      w322 = T8 1 items=["FEATURE_FLAG_PRESENCE                 0x00000001", "FEATURE_FLAG_MANUAL                     0x00000002", "FEATURE_FLAG_AUTO                         0x00000004", "FEATURE_FLAG_ONEPUSH                   0x00000008", "FEATURE_FLAG_OFF                            0x00000010", "FEATURE_FLAG_DESC_SUPPORTED    0x00000020", "FEATURE_FLAG_READ_ONLY               0x00000040"] ("uFlags IN")
                      w323 = T9 0 items=["FEATURE_BRIGHTNESS", "FEATURE_EXPOSURE", "FEATURE_SHARPNESS", "FEATURE_WHITE_BAL", "FEATURE_HUE", "FEATURE_SATURATION", "FEATURE_GAMMA", "FEATURE_SHUTTER", "FEATURE_GAIN", "FEATURE_IRIS", "FEATURE_FOCUS", "FEATURE_TEMPERATURE", "FEATURE_TRIGGER", "FEATURE_ZOOM", "FEATURE_PAN", "FEATURE_TILT", "FEATURE_OPT_FILTER", "FEATURE_GPIO", "FEATURE_FRAME_RATE", "FEATURE_ROI", "FEATURE_FLIP", "FEATURE_PIXEL_ADDRESSING", "FEATURE_PIXEL_FORMAT", "FEATURE_EXTENDED_SHUTTER", "FEATURE_AUTO_ROI", "FEATURE_LOOKUP_TABLE", "FEATURE_MEMORY_CHANNEL", "FEATURE_WHITE_SHADING", "FEATURE_ROTATE", "FEATURE_IMAGER_CLK_DIVISOR", "FEATURE_TRIG_WITH_CNTRLD_LIGHT", "FEATURE_MAX_PIXEL_SIZE"] ("uFeatureId IN")
                      n101 = call <vilib>:"MEPU-CameraFeatures-SetFeature.vi"("hCamera IN"=w325, "uFeatureId IN"=w323, "uFlags IN"=w322, "pParms IN"=w317, "Error IN"=w324) -> ("hCamera OUT"=w321:u32, "Error OUT"=w316:errorcluster)  [unwired: 8 in, 1 out]
                      n102 = call "showError.vi"("message"="Ocurrio un error con el Brightness", "Error IN"=w316) -> ("Error OUT"=w315:errorcluster)  [unwired: 3 in]
                      n103 = call "getCameraParameters.vi"("Error IN"=w315, "hCamera IN"=w321) -> ("Error OUT"=w319:errorcluster, "Camera Parameters"=w318:T6, "hCamera OUT"=w320:u32)  [unwired: 1 in]
                      n104 = call "StartStopCamera.vi"("Error IN"=w319, "Camara ON?"=w328, "hCamera IN"=w320) -> ("Error OUT"=w326:errorcluster, "hCamera OUT"=w327:u32)  [unwired: 1 in]
                    }
                  }
                  n105 = Unbundle By Name(w302) -> ("Stream?"=w304:bool, "Camera Parameters.Brightness (%)"=w301:dbl)
                  n106 = Build Array(w301) -> (w298:dbl[])
                  n107 = To Double Precision Float(number=w298) -> (double precision float=w297:dbl[])
                  n108 = Bundle By Name(cluster=w302, "Camera Parameters"=w300) -> (w303:T4)
                  n109 = call "camera2cluster.vi"("uSerialNumber IN"=w292, "Error IN"=w295, "hCamera IN"=w296) -> ("Camera Device OUT"=w294:T1)
                }
                frame "Pixel Format" {
                  n110 = call "cluster2camera.vi"("Camera Device IN"=w330) -> ("Error OUT"=w342:errorcluster, "hCamera OUT"=w343:u32, "uSerialNumber OUT"=w329:u32)  [unwired: 2 in]
                  n111 = flat-sequence {
                    tunnel: w343 -> [w349]
                    tunnel: w342 -> [w348]
                    tunnel: [w347] -> w345
                    tunnel: [w346] -> w344
                    tunnel: w339 -> [w365]
                    tunnel: [w364] -> w341
                    tunnel: [w363] -> w340
                    tunnel: w345 -> [w362]
                    tunnel: w344 -> [w361]
                    tunnel: [w355] -> w335
                    tunnel: w332 -> [w354]
                    frame #0 {
                      n112 = call "StartStopCamera.vi"("Error IN"=w348, "Camara ON?"=FALSE, "hCamera IN"=w349) -> ("Error OUT"=w346:errorcluster, "hCamera OUT"=w347:u32)  [unwired: 1 in]
                    }
                    frame #1 {
                      w359 = T8 1 items=["FEATURE_FLAG_PRESENCE                 0x00000001", "FEATURE_FLAG_MANUAL                     0x00000002", "FEATURE_FLAG_AUTO                         0x00000004", "FEATURE_FLAG_ONEPUSH                   0x00000008", "FEATURE_FLAG_OFF                            0x00000010", "FEATURE_FLAG_DESC_SUPPORTED    0x00000020", "FEATURE_FLAG_READ_ONLY               0x00000040"] ("uFlags IN")
                      w360 = T9 22 items=["FEATURE_BRIGHTNESS", "FEATURE_EXPOSURE", "FEATURE_SHARPNESS", "FEATURE_WHITE_BAL", "FEATURE_HUE", "FEATURE_SATURATION", "FEATURE_GAMMA", "FEATURE_SHUTTER", "FEATURE_GAIN", "FEATURE_IRIS", "FEATURE_FOCUS", "FEATURE_TEMPERATURE", "FEATURE_TRIGGER", "FEATURE_ZOOM", "FEATURE_PAN", "FEATURE_TILT", "FEATURE_OPT_FILTER", "FEATURE_GPIO", "FEATURE_FRAME_RATE", "FEATURE_ROI", "FEATURE_FLIP", "FEATURE_PIXEL_ADDRESSING", "FEATURE_PIXEL_FORMAT", "FEATURE_EXTENDED_SHUTTER", "FEATURE_AUTO_ROI", "FEATURE_LOOKUP_TABLE", "FEATURE_MEMORY_CHANNEL", "FEATURE_WHITE_SHADING", "FEATURE_ROTATE", "FEATURE_IMAGER_CLK_DIVISOR", "FEATURE_TRIG_WITH_CNTRLD_LIGHT", "FEATURE_MAX_PIXEL_SIZE"] ("uFeatureId IN")
                      n113 = call <vilib>:"MEPU-CameraFeatures-SetFeature.vi"("hCamera IN"=w362, "uFeatureId IN"=w360, "uFlags IN"=w359, "pParms IN"=w354, "Error IN"=w361) -> ("hCamera OUT"=w358:u32, "Error OUT"=w353:errorcluster)  [unwired: 8 in, 1 out]
                      n114 = call "showError.vi"("message"="Ocurrio un error con el Pixel Format", "Error IN"=w353) -> ("Error OUT"=w352:errorcluster)  [unwired: 3 in]
                      n115 = call "getCameraParameters.vi"("Error IN"=w352, "hCamera IN"=w358) -> ("Error OUT"=w356:errorcluster, "Camera Parameters"=w355:T6, "hCamera OUT"=w357:u32)  [unwired: 1 in]
                      n116 = call "StartStopCamera.vi"("Error IN"=w356, "Camara ON?"=w365, "hCamera IN"=w357) -> ("Error OUT"=w363:errorcluster, "hCamera OUT"=w364:u32)  [unwired: 1 in]
                    }
                  }
                  n117 = Unbundle By Name(w337) -> ("Stream?"=w339:bool, "Camera Parameters.Pixel Format"=w336:T3)
                  n118 = Build Array(w336) -> (w333:T3[])
                  n119 = To Double Precision Float(number=w333) -> (double precision float=w332:dbl[])
                  n120 = Bundle By Name(cluster=w337, "Camera Parameters"=w335) -> (w338:T4)
                  n121 = call "camera2cluster.vi"("uSerialNumber IN"=w329, "Error IN"=w340, "hCamera IN"=w341) -> ("Camera Device OUT"=w331:T1)
                }
                frame "Color Temperature (%)" {
                  n122 = call "cluster2camera.vi"("Camera Device IN"=w368) -> ("Error OUT"=w379:errorcluster, "hCamera OUT"=w380:u32, "uSerialNumber OUT"=w367:u32)  [unwired: 2 in]
                  n123 = Unbundle By Name(w374) -> ("Stream?"=w376:bool, "Camera Parameters.Color Temperature"=w373:dbl)
                  n124 = flat-sequence {
                    tunnel: w380 -> [w386]
                    tunnel: w379 -> [w385]
                    tunnel: [w384] -> w382
                    tunnel: [w383] -> w381
                    tunnel: w376 -> [w402]
                    tunnel: [w401] -> w378
                    tunnel: [w400] -> w377
                    tunnel: w382 -> [w399]
                    tunnel: w381 -> [w398]
                    tunnel: [w392] -> w372
                    tunnel: w369 -> [w391]
                    frame #0 {
                      n125 = call "StartStopCamera.vi"("Error IN"=w385, "Camara ON?"=FALSE, "hCamera IN"=w386) -> ("Error OUT"=w383:errorcluster, "hCamera OUT"=w384:u32)  [unwired: 1 in]
                    }
                    frame #1 {
                      w396 = T8 1 items=["FEATURE_FLAG_PRESENCE                 0x00000001", "FEATURE_FLAG_MANUAL                     0x00000002", "FEATURE_FLAG_AUTO                         0x00000004", "FEATURE_FLAG_ONEPUSH                   0x00000008", "FEATURE_FLAG_OFF                            0x00000010", "FEATURE_FLAG_DESC_SUPPORTED    0x00000020", "FEATURE_FLAG_READ_ONLY               0x00000040"] ("uFlags IN")
                      w397 = T9 11 items=["FEATURE_BRIGHTNESS", "FEATURE_EXPOSURE", "FEATURE_SHARPNESS", "FEATURE_WHITE_BAL", "FEATURE_HUE", "FEATURE_SATURATION", "FEATURE_GAMMA", "FEATURE_SHUTTER", "FEATURE_GAIN", "FEATURE_IRIS", "FEATURE_FOCUS", "FEATURE_TEMPERATURE", "FEATURE_TRIGGER", "FEATURE_ZOOM", "FEATURE_PAN", "FEATURE_TILT", "FEATURE_OPT_FILTER", "FEATURE_GPIO", "FEATURE_FRAME_RATE", "FEATURE_ROI", "FEATURE_FLIP", "FEATURE_PIXEL_ADDRESSING", "FEATURE_PIXEL_FORMAT", "FEATURE_EXTENDED_SHUTTER", "FEATURE_AUTO_ROI", "FEATURE_LOOKUP_TABLE", "FEATURE_MEMORY_CHANNEL", "FEATURE_WHITE_SHADING", "FEATURE_ROTATE", "FEATURE_IMAGER_CLK_DIVISOR", "FEATURE_TRIG_WITH_CNTRLD_LIGHT", "FEATURE_MAX_PIXEL_SIZE"] ("uFeatureId IN")
                      n126 = call <vilib>:"MEPU-CameraFeatures-SetFeature.vi"("hCamera IN"=w399, "uFeatureId IN"=w397, "uFlags IN"=w396, "pParms IN"=w391, "Error IN"=w398) -> ("hCamera OUT"=w395:u32, "Error OUT"=w390:errorcluster)  [unwired: 8 in, 1 out]
                      n127 = call "showError.vi"("message"="Ocurrio un error con el Coor Tenperature", "Error IN"=w390) -> ("Error OUT"=w389:errorcluster)  [unwired: 3 in]
                      n128 = call "getCameraParameters.vi"("Error IN"=w389, "hCamera IN"=w395) -> ("Error OUT"=w393:errorcluster, "Camera Parameters"=w392:T6, "hCamera OUT"=w394:u32)  [unwired: 1 in]
                      n129 = call "StartStopCamera.vi"("Error IN"=w393, "Camara ON?"=w402, "hCamera IN"=w394) -> ("Error OUT"=w400:errorcluster, "hCamera OUT"=w401:u32)  [unwired: 1 in]
                    }
                  }
                  n130 = Build Array(w373) -> (w370:dbl[])
                  n131 = To Double Precision Float(number=w370) -> (double precision float=w369:dbl[])
                  n132 = Bundle By Name(cluster=w374, "Camera Parameters"=w372) -> (w375:T4)
                  n133 = call "camera2cluster.vi"("uSerialNumber IN"=w367, "Error IN"=w377, "hCamera IN"=w378) -> ("Camera Device OUT"=w366:T1)
                }
                frame "Selector" {
                  n134 = Unbundle By Name(w415) -> ("Selector"=w408:u16, "Stream?"=w407:bool)
                  n135 = call "cluster2camera.vi"("Camera Device IN"=w405) -> ("Error OUT"=w413:errorcluster, "hCamera OUT"=w414:u32, "uSerialNumber OUT"=w403:u32)  [unwired: 2 in]
                  n136 = flat-sequence {
                    tunnel: w414 -> [w418]
                    tunnel: w413 -> [w417]
                    tunnel: w406 -> [w428]
                    tunnel: [w424] -> w410
                    tunnel: w407 -> [w423]
                    tunnel: [w421] -> w412
                    tunnel: [w420] -> w411
                    frame #0 {
                      n137 = call "StartStopCamera.vi"("Error IN"=w417, "Camara ON?"=FALSE, "hCamera IN"=w418) -> ()  [unwired: 1 in, 2 out]
                    }
                    frame #1 {
                      n138 = call <vilib>:"MEPU-Initialization-Initialize.vi"("uSerialNumber IN"=w428) -> ("phCamera OUT"=w427:u32, "Error OUT"=w426:errorcluster)  [unwired: 12 in, 1 out]
                      n139 = call "getCameraParameters.vi"("Error IN"=w426, "hCamera IN"=w427) -> ("Error OUT"=w425:errorcluster, "Camera Parameters"=w424:T6, "hCamera OUT"=w422:u32)  [unwired: 1 in]
                      n140 = call "StartStopCamera.vi"("Error IN"=w425, "Camara ON?"=w423, "hCamera IN"=w422) -> ("Error OUT"=w420:errorcluster, "hCamera OUT"=w421:u32)  [unwired: 1 in]
                    }
                  }
                  n141 = Index Array(array=w409, index=w408) -> (element=w406:u32)
                  n142 = Bundle By Name(cluster=w415, "Camera Parameters"=w410) -> (w416:T4)
                  n143 = call "camera2cluster.vi"("uSerialNumber IN"=w403, "Error IN"=w411, "hCamera IN"=w412) -> ("Camera Device OUT"=w404:T1)
                }
                frame "Stream" {
                  n144 = Unbundle By Name(w437) -> ("Stream?"=w432:bool)
                  n145 = call "cluster2camera.vi"("Camera Device IN"=w431) -> ("Error OUT"=w435:errorcluster, "hCamera OUT"=w436:u32, "uSerialNumber OUT"=w429:u32)  [unwired: 2 in]
                  n146 = call "StartStopCamera.vi"("Error IN"=w435, "Camara ON?"=w432, "hCamera IN"=w436) -> ("Error OUT"=w433:errorcluster, "hCamera OUT"=w434:u32)  [unwired: 1 in]
                  n147 = call "camera2cluster.vi"("uSerialNumber IN"=w429, "Error IN"=w433, "hCamera IN"=w434) -> ("Camera Device OUT"=w430:T1)
                }
                frame "Nothing", Default {
                }
              }
            }
          }
        }
      }
    }
  }
  "Camera Device OUT" <- w1
  n148 = Unbundle By Name(w12) -> ("Camera Parameters"=w11:T5, "Stream?"=w5:bool)
  "Stream? OUT" <- w5
  n149 = property class="Clust (strict)"(reference="Camera Parameters", "Value"=w11) -> ()  [unwired: 1 in, 2 out]
  n150 = property class="Bool (strict)"(reference="Stream?", "Value"=w5) -> ()  [unwired: 1 in, 2 out]
